vi "Exemple_Preprocessing_Normalizer.vi"() -> ()   [LabVIEW 2020]
uses:
  Objet/6 - Datasets Transformation/6.3 - Processing Data/Normalizer/Normalizer.lvclass
panel:
  in  "y":string[][](array[string])
  in  "X":string[][](array[string])=[["4", "1", "2", "2"], ["1", "3", "9", "3"], ["5", "7", "5", "1"]]
  out "Data":T1
  out "error out":errorcluster
  in  "error in":errorcluster caption="entrée d'erreur"
  in  "Normalizer":cluster{"norm":string, "copy":bool}={"norm"="l2", "copy"=TRUE}
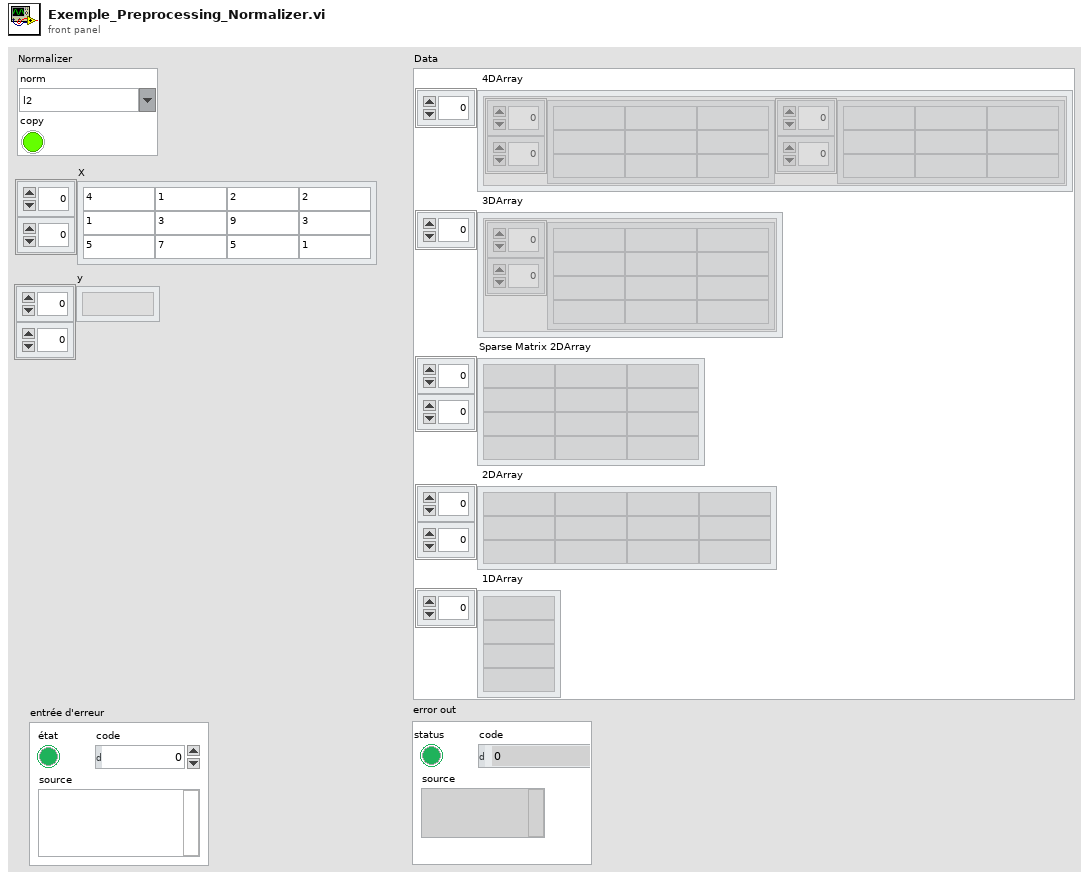
[diagram p1: front panel]
types:
  T1 = cluster{" 4DArray":cluster{"1":string[][], "2":string[][]}[], " 3DArray":cluster{"Tableau":string[][]}[], "Sparse Matrix 2DArray":string[][], " 2DArray":string[][], " 1DArray":string[]}
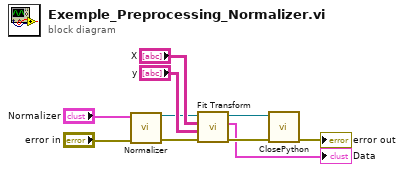
[diagram p0: block diagram]
diagram:
  n1 = call "Normalizer.vi"("error in (no error)"="error in", "Normalizer"="Normalizer") -> ("error out"=w8:errorcluster, "Normalizer.lvclass"=w5:refnum<class "Normalizer.lvclass">)  [unwired: 8 in]
  n2 = call-dynamic "Fit Transform.vi"("error in (no error)"=w8, "y"="y", "X"="X", "Normalizer.lvclass"=w5) -> ("error out"=w3:errorcluster, "Data"=→"Data":T1, "Normalizer.lvclass"=w4:refnum<class "Normalizer.lvclass">)  [unwired: 5 in]
  n3 = call-dynamic "ClosePython.vi"("error in (no error)"=w3, "Scikit-learn en entrée"=w4) -> ("error out"=→"error out":errorcluster)  [unwired: 8 in, 1 out]
